vi "Door Switch.vi"(8 "error in (no error)":errorcluster) -> (0 "error out":errorcluster, 3 "Door Switch Activation":i16)   [LabVIEW 2012]
uses:
  <vilib>/DAQmx/read.llb/DAQmx Read (Digital 1D Bool NChan 1Samp 1Line).vi
  <vilib>/DAQmx/miscellaneous.llb/DAQmx Fill In Error Info.vi
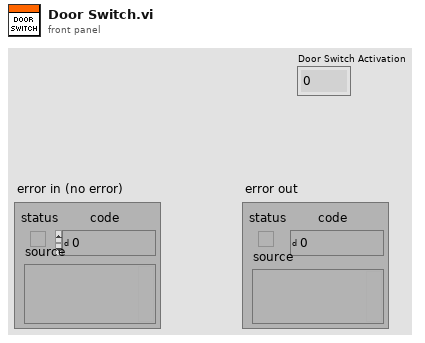
[diagram p1: front panel]
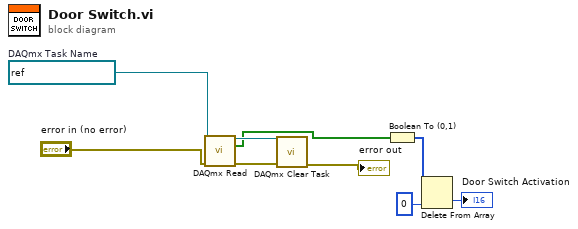
[diagram p0: block diagram]
diagram:
  w7 = refnum<k21> "DoorSwitch"  # DAQmx Task Name
  n1 = call-poly <vilib>:"DAQmx Read.vi"("task/channels in"=w7, "error in"="error in (no error)") -> ("task out"=w8:refnum<k21>, "data"=w6:bool[], "error out"=w9:errorcluster)  [unwired: 1 in, 10 out]
  n2 = call <vilib>:"DAQmx Clear Task.vi"("task in"=w8, "error in"=w9) -> ("error out"=→"error out":errorcluster)  [unwired: 13 out]
  n3 = Boolean To (0,1)(Boolean=w6) -> (0, 1=w5:i16[])
  n4 = Delete From Array(array=w5, index=0) -> (deleted portion=→"Door Switch Activation":i16)  [unwired: 1 in, 1 out]
